vi "init.vi"(8 "error in (no error)":errorcluster, 11 "ATDomeCommunicator in":refnum<class "ATDomeCommunicator.lvclass">) -> (0 "error out":errorcluster, 3 "ATDomeCommunicator out":refnum<class "ATDomeCommunicator.lvclass">)   [LabVIEW 2016, in "ATDomeCommunicator.lvclass"]
uses:
  ATDomeCommunicator.lvclass
  home/plotz/lsst_ts/ss_atDome/common_labview_tcpdevice/tcpDevice/tcpDevice.lvclass
  common_labview_tcpdevice/tcpDevice/tcpDevice.lvclass
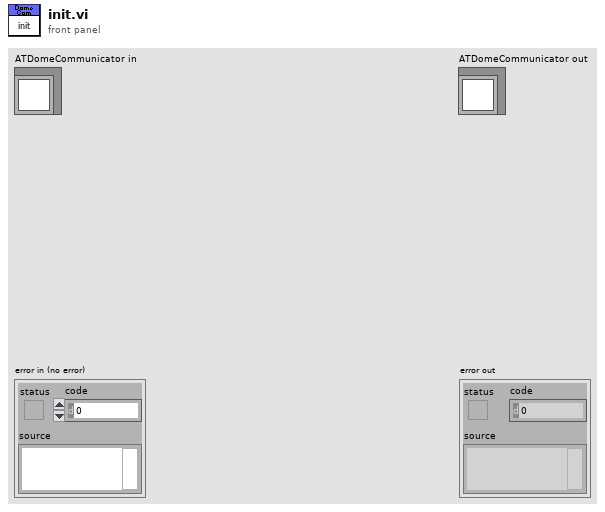
[diagram p1: front panel]
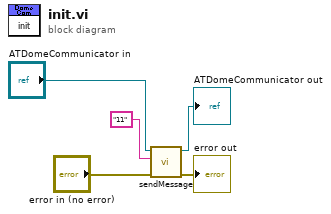
[diagram p0: block diagram]
diagram:
  n1 = call "sendMessage.vi"("error in (no error)"="error in (no error)", "Message"="11", "tcpDevice in"="ATDomeCommunicator in") -> ("error out"=→"error out":errorcluster, "tcpDevice out"=→"ATDomeCommunicator out":refnum<class "ATDomeCommunicator.lvclass">)  [unwired: 7 in]
